vi "inverse calibration function CO2.vi"(7 "x":dbl format="%#_13g") -> (8 "f_inv(x)":dbl)   [LabVIEW 2017, in "LicorLI7000.lvlib"]
uses:
  LicorLI7000.lvlib
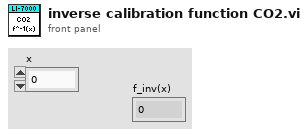
[diagram p1: front panel]
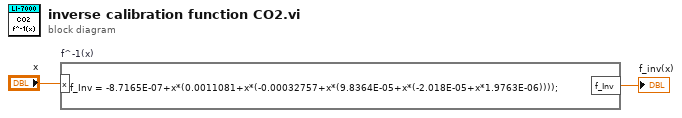
[diagram p0: block diagram]
diagram:
  n1 = formula code="f_Inv = -8.7165E-07+x*(0.0011081+x*(-0.00032757+x*(9.8364E-05+x*(-2.018E-05+x*1.9763E-06))));" "f^-1(x)"("x"="x") -> ("f_Inv"=→"f_inv(x)":dbl)
